vi "API_Call.vi"(6 "Server":path, 7 "Direction":enum16{"ASK", "TELL"}(ring), 8 "error in (no error)":errorcluster, 9 "Payload":string, 11 "cmd":string) -> (0 "error out":errorcluster, 1 "Running?":bool, 2 "Send to Server":string, 3 "Read from Server":string)   [LabVIEW 2020]
uses:
  JSON_Formats.vi
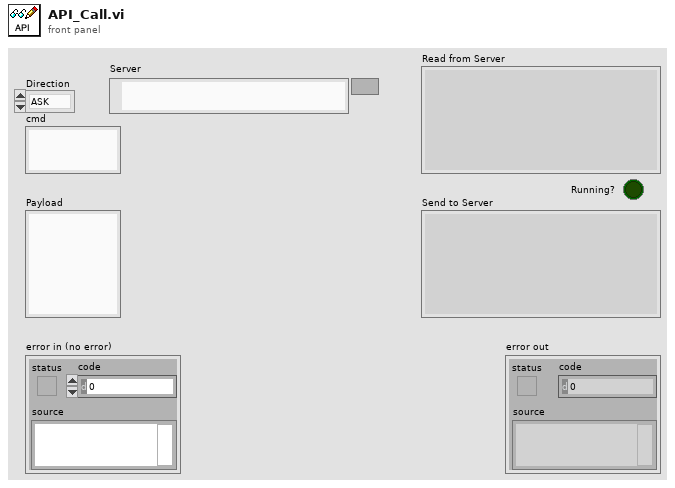
[diagram p1: front panel]
types:
  T1 = enum32{"Bad", "Idle", "Run top level", "Running"}
  T2 = enum32{"Invalid", "Standard", "Closed", "Hidden", "Minimized", "Maximized"}
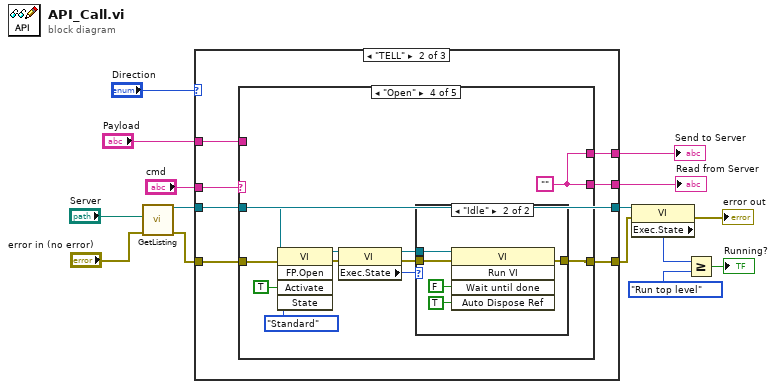
[diagram p0: block diagram]
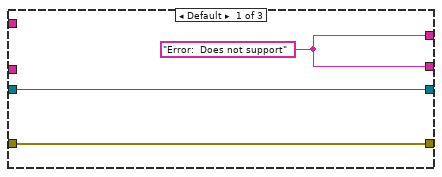
[diagram p2: hidden frame]
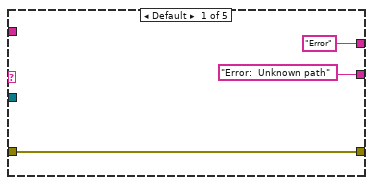
[diagram p3: hidden frame]
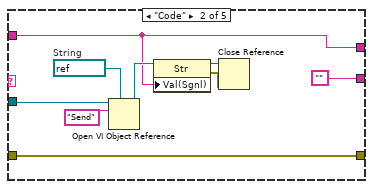
[diagram p4: hidden frame]
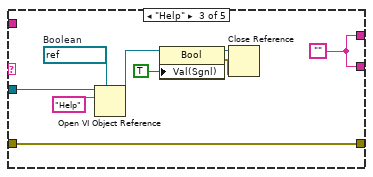
[diagram p5: hidden frame]
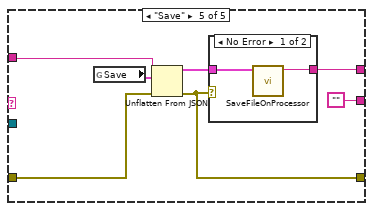
[diagram p7: hidden frame]
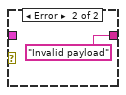
[diagram p8: hidden frame]
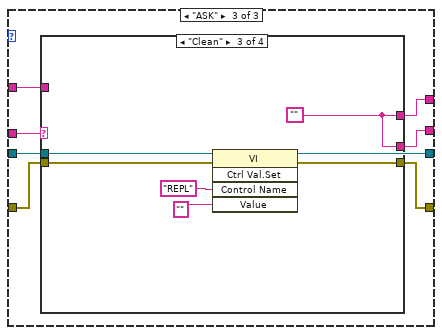
[diagram p9: hidden frame]
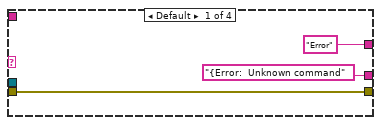
[diagram p10: hidden frame]
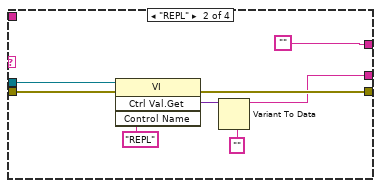
[diagram p11: hidden frame]
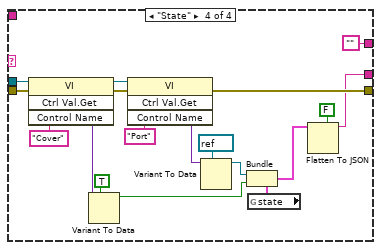
[diagram p12: hidden frame]
diagram:
  n1 = call "GetListing.vi"("error in (no error)"="error in (no error)", "Server"="Server") -> ("error out"=w7:errorcluster, "VI out"=w12:refnum<vi>)  [unwired: 8 in]
  n2 = case shown="\"TELL\"" "Direction" {
    tunnel: [w18 w25 w80] -> w15
    tunnel: "Payload" -> [_ w24 w79]
    tunnel: [w18 w23 w78] -> w14
    tunnel: w12 -> [w16 w19 w74]
    tunnel: w7 -> [w17 w22 w77]
    tunnel: [w17 w21 w76] -> w5
    tunnel: "cmd" -> [_ w20 w75]
    tunnel: [w16 w19 w74] -> w6
    frame Default {
      w18 = "Error:  Does not support" ("input 2")
    }
    frame "TELL" {
      n3 = case shown="\"Open\"" w20 {
        tunnel: ["Error:  Unknown path" ("input 2") "" w38 w55 ""] -> w25
        tunnel: w24 -> [_ w31 _ _ w70]
        tunnel: ["Error" ("input 2") w31 w38 w55 w68] -> w23
        tunnel: w22 -> [w26 w36 w46 w53 w66]
        tunnel: [w26 w36 w46 w47 w65] -> w21
        tunnel: w19 -> [_ w33 w43 w54 _]
        frame Default {
        }
        frame "Code" {
          w35 = refnum<vi> refnum  # String
          n4 = Open VI Object Reference(7:w35, 10:"Send" ("name/order"), 11:w33) -> (3:w32:refnum<vi>)  [unwired: 1 in, 1 out]
          n5 = property class="Str"(reference=w32, "Val(Sgnl)"=w31) -> (reference out=w29:refnum<vi>, error out=w30:errorcluster)  [unwired: 1 in]
          n6 = Close Reference(reference=w29, error in (no error)=w30) -> ()  [unwired: 1 out]
        }
        frame "Help" {
          w45 = refnum<vi> refnum  # Boolean
          w38 = ""
          n7 = Open VI Object Reference(7:w45, 10:"Help" ("name/order"), 11:w43) -> (3:w42:refnum<vi>)  [unwired: 1 in, 1 out]
          n8 = property class="Bool"(reference=w42, "Val(Sgnl)"=TRUE) -> (reference out=w40:refnum<vi>, error out=w41:errorcluster)  [unwired: 1 in]
          n9 = Close Reference(reference=w40, error in (no error)=w41) -> ()  [unwired: 1 out]
        }
        frame "Open" {
          w55 = ""
          n10 = invoke class="VI" method="FP.Open"(reference=w54, error in=w53, "Activate"=TRUE ("Activate?"), "State"=T2."Standard" ("Front Panel Window:State")) -> (reference out=w52:refnum<vi>, error out=w51:errorcluster)  [unwired: 1 in, 3 out]
          n11 = property class="VI"(reference=w52, error in=w51) -> (reference out=w49:refnum<vi>, error out=w48:errorcluster, "Exec.State"=w50:T1)
          n12 = case shown="\"Idle\"" w50 {
            tunnel: w49 -> [_ w63]
            tunnel: w48 -> [w58 w62]
            tunnel: [w58 w61] -> w47
            frame Default {
            }
            frame "Idle" {
              n13 = invoke class="VI" method="Run VI"(reference=w63, error in=w62, "Wait until done"=FALSE ("Activate?"), "Auto Dispose Ref"=TRUE ("Activate?")) -> (error out=w61:errorcluster)  [unwired: 1 in, 4 out]
            }
          }
        }
        frame "Save" {
          n14 = global read "JSON_Formats.vi" "Save"() -> (w67:cluster{"fileName":string, "Code":string})
          n15 = Unflatten From JSON(JSON string=w70, type and defaults=w67, error in (no error)=w66) -> (value=w69:cluster{"fileName":string, "Code":string}, error out=w65:errorcluster)  [unwired: 4 in]
          n16 = case shown="No Error" w65 {
            tunnel: w69 -> [w72 _]
            tunnel: [w71 "Invalid payload" ("Code")] -> w68
            frame No Error {
              n17 = call "SaveFileOnProcessor.vi"("Save"=w72) -> ("Code"=w71:string)  [unwired: 10 in]
            }
            frame Error {
            }
          }
        }
      }
    }
    frame "ASK" {
      n18 = case shown="\"Clean\"" w75 {
        tunnel: ["{Error:  Unknown command" ("input 2") w84 w97 w98] -> w80
        tunnel: w79 -> [_ _ _ _]
        tunnel: ["Error" ("input 2") "" w97 ""] -> w78
        tunnel: w74 -> [_ w86 w94 w108]
        tunnel: w77 -> [w81 w87 w93 w107]
        tunnel: [w81 w85 w92 w104] -> w76
        frame Default {
        }
        frame "REPL" {
          n19 = invoke class="VI" method="Ctrl Val.Get"(reference=w86, error in=w87, "Control Name"="REPL") -> (error out=w85:errorcluster, "Get Control Value Variant"=w89:variant)  [unwired: 1 in, 2 out]
          n20 = Variant To Data(type="" ("Control Name"), Variant=w89) -> (data=w84:string)  [unwired: 1 in, 1 out]
        }
        frame "Clean" {
          w97 = ""
          n21 = invoke class="VI" method="Ctrl Val.Set"(reference=w94, error in=w93, "Control Name"="REPL", "Value"="" ("Control Name")) -> (error out=w92:errorcluster)  [unwired: 1 in, 4 out]
        }
        frame "State" {
          n22 = invoke class="VI" method="Ctrl Val.Get"(reference=w108, error in=w107, "Control Name"="Cover") -> (reference out=w106:refnum<vi>, error out=w105:errorcluster, "Get Control Value Variant"=w109:variant)  [unwired: 1 in, 1 out]
          n23 = Variant To Data(type=TRUE, Variant=w109) -> (data=w102:bool)  [unwired: 1 in, 1 out]
          n24 = invoke class="VI" method="Ctrl Val.Get"(reference=w106, error in=w105, "Control Name"="Port") -> (error out=w104:errorcluster, "Get Control Value Variant"=w110:variant)  [unwired: 1 in, 2 out]
          n25 = Variant To Data(type=refnum<visa-resource-name> refnum ("Port"), Variant=w110) -> (data=w103:refnum<visa-resource-name>)  [unwired: 1 in, 1 out]
          n26 = global read "JSON_Formats.vi" "state"() -> (w101:cluster{"Connection":string, "Connected?":bool})
          n27 = Bundle(cluster=w101, "Connection"=w103, "Connected?"=w102) -> (w100:cluster{"Connection":string, "Connected?":bool})
          n28 = Flatten To JSON(enable LabVIEW extensions? (T)=FALSE, anything=w100) -> (JSON string=w98:string)  [unwired: 1 in, 1 out]
        }
      }
    }
  }
  "Read from Server" <- w15
  "Send to Server" <- w14
  n29 = property class="VI"(reference=w6, error in=w5) -> (error out=→"error out":errorcluster, "Exec.State"=w4:T1)  [unwired: 1 out]
  n30 = Greater Or Equal?(x=w4, y=T1."Run top level" ("Execution:State")) -> (x >= y?=→"Running?":bool)
